vi "DROP TABLE IF EXISTS.vi"(8 "error in (no error)":errorcluster, 11 "ORM Scripter in":refnum<class "ORM Scripter.lvclass">) -> (0 "error out":errorcluster, 1 "Drop if exists":string, 3 "ORM Scripter OUT":refnum<class "ORM Scripter.lvclass">)   [LabVIEW 2018, in "ORM Scripter.lvclass"]
uses:
  ORM Scripter.lvclass
  ORM Scripter.lvclass/ORM Scripter.ctl
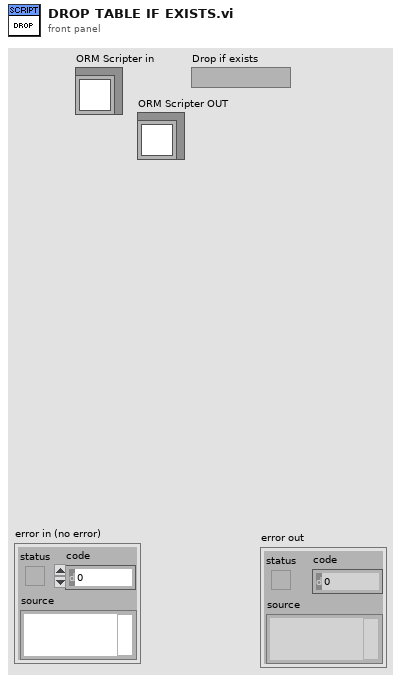
[diagram p1: front panel]
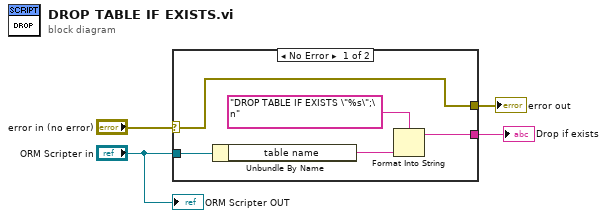
[diagram p0: block diagram]
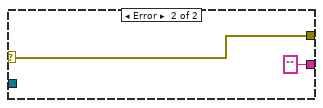
[diagram p2: hidden frame]
diagram:
  n1 = case shown="No Error" "error in (no error)" {
    selector: "error in (no error)" -> [w6 w11]
    tunnel: [w6 w11] -> w4
    tunnel: "ORM Scripter in" -> [w7 _]
    tunnel: [w5 ""] -> w1
    frame No Error {
      n2 = Unbundle By Name(w7) -> ("table name"=w9:string)
      n3 = Format Into String(format string="DROP TABLE IF EXISTS \"%s\";\n", w9) -> (resulting string=w5:string)  [unwired: 2 in, 1 out]
    }
    frame Error {
    }
  }
  "error out" <- w4
  "Drop if exists" <- w1
  "ORM Scripter OUT" <- "ORM Scripter in"
